vi "SetSyncSettings.vi"(6 "X SyncOut Enabled":bool=TRUE, 7 "Y SyncOut Enabled":bool, 8 "error in (no error)":errorcluster, 9 "Calibration":cluster{dbl, "MicrostepMode":u32}[](array[cluster]), 10 "Step Sizes(mm)":dbl[](array[numeric]), 11 "IDs":i32[](array[numeric])) -> (0 "error out":errorcluster, 3 "IDs Out":i32[](array[numeric]))   [LabVIEW 2020]
uses:
  Sync_outFlags.ctl
  Sync_inFlags.ctl
  libximc.lvlib
panel:
  out "SyncOutPeriod":u32[](array[numeric])
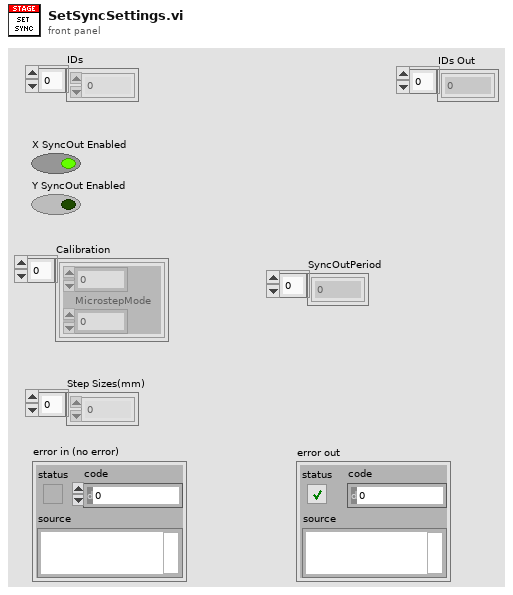
[diagram p1: front panel]
types:
  T1 = cluster{"SyncInFlags":u32, "ClutterTime":u32, "Position":sgl, "Speed":sgl}
  T2 = typedef "Sync_inFlags.ctl" = cluster{"Enabled":bool, "invert":bool, "go_to_position":bool}
  T3 = cluster{"SyncOutFlags":u32, "SyncOutPulseSteps":u32, "SyncOutPeriod":u32, "Accuracy":sgl}
  T4 = typedef "Sync_outFlags.ctl" = cluster{"Enabled":bool, "state":bool, "invert":bool, "in_steps":bool, "on_start":bool, "on_stop":bool, "on_period":bool}
  T5 = cluster{"SyncInFlags":u32, "ClutterTime":u32, "Position":sgl, "Speed":sgl}[]
  T6 = cluster{"SyncOutFlags":u32, "SyncOutPulseSteps":u32, "SyncOutPeriod":u32, "Accuracy":sgl}[]
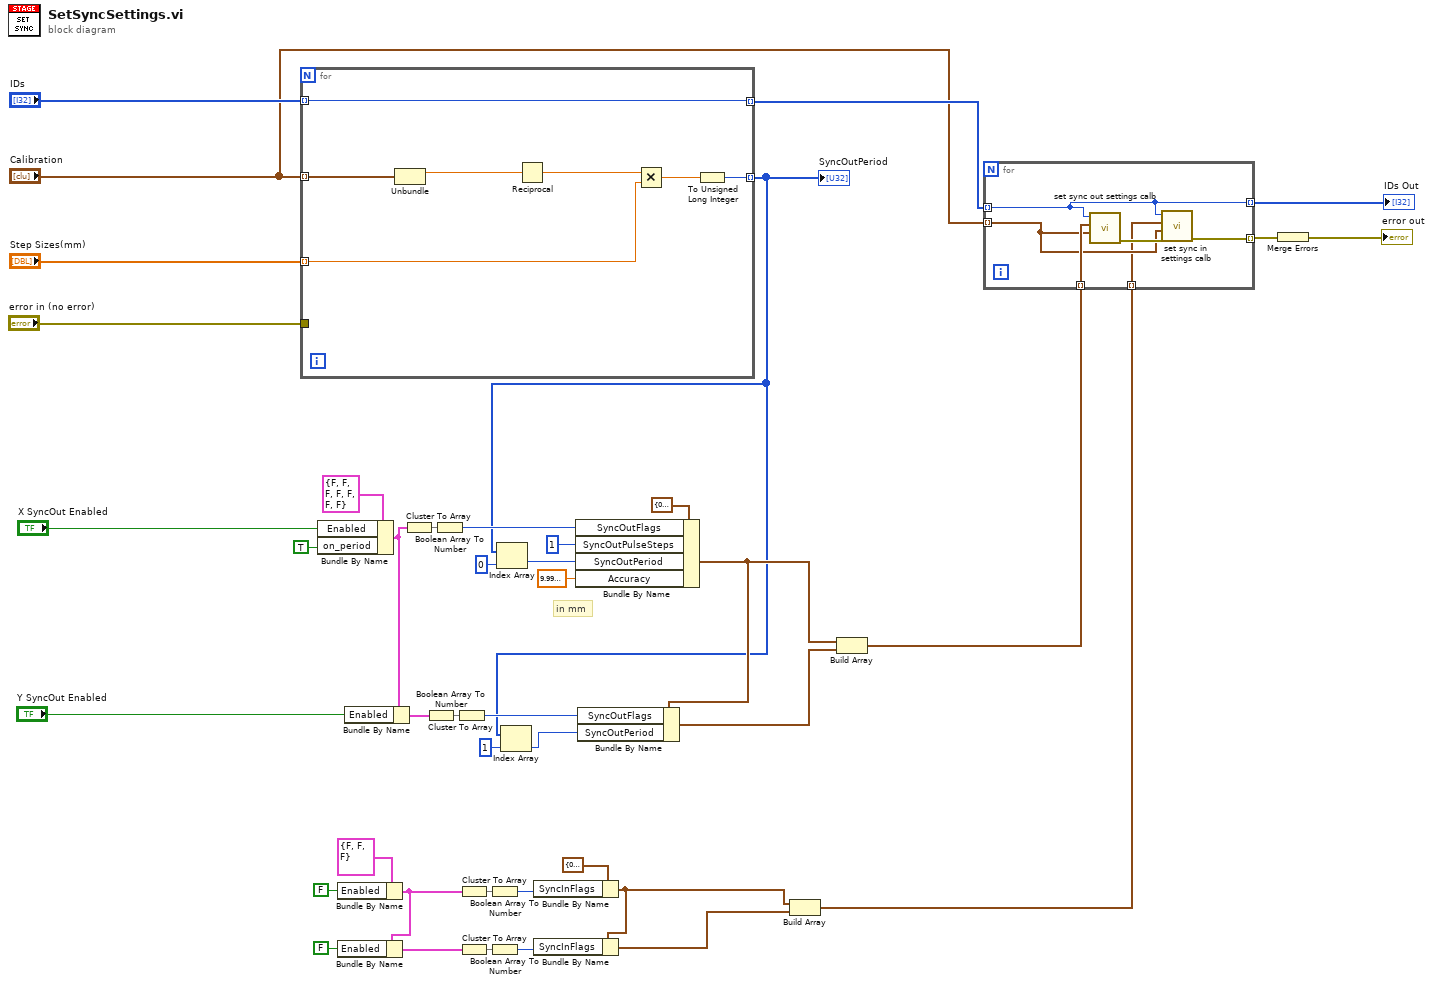
[diagram p0: block diagram]
diagram:
  # "in mm"
  n1 = for {
    tunnel: [w49] -> w21 mode=indexing
    tunnel: "IDs" -> [w49] mode=indexing
    tunnel: "Calibration" -> [w48] mode=indexing
    tunnel: "Step Sizes(mm)" -> [w47] mode=indexing
    tunnel: [w46] -> w22 mode=indexing
    tunnel: "error in (no error)" -> [_]
    n2 = Unbundle(w48) -> (w45:dbl)  [unwired: 1 out]
    n3 = Reciprocal(x=w45) -> (1/x=w44:dbl)
    n4 = Multiply(x=w44, y=w47) -> (x*y=w43:dbl)
    n5 = To Unsigned Long Integer(number=w43) -> (unsigned 32bit integer=w46:u32)
  }
  "SyncOutPeriod" <- w22
  n6 = Bundle By Name(cluster=T4 {"Enabled"=FALSE, "state"=FALSE, "invert"=FALSE, "in_steps"=FALSE, "on_start"=FALSE, "on_stop"=FALSE, "on_period"=FALSE} ("Sync_out Flags"), "Enabled"="X SyncOut Enabled", "on_period"=TRUE) -> (w27:T4)
  n7 = Bundle By Name(cluster=T2 {"Enabled"=FALSE, "invert"=FALSE, "go_to_position"=FALSE} ("Sync_out Flags"), "Enabled"=FALSE) -> (w7:T2)
  n8 = Bundle By Name(cluster=w7, "Enabled"=FALSE) -> (w8:T2)
  n9 = Bundle By Name(cluster=w27, "Enabled"="Y SyncOut Enabled") -> (w35:T4)
  n10 = Cluster To Array(cluster=w27) -> (array=w40:bool[])
  n11 = Cluster To Array(cluster=w35) -> (array=w36:bool[])
  n12 = Boolean Array To Number(Boolean array=w40) -> (number=w39:u32)
  n13 = Boolean Array To Number(Boolean array=w36) -> (number=w37:u32)
  n14 = Cluster To Array(cluster=w7) -> (array=w18:bool[])
  n15 = Cluster To Array(cluster=w8) -> (array=w9:bool[])
  n16 = Boolean Array To Number(Boolean array=w18) -> (number=w17:u32)
  n17 = Boolean Array To Number(Boolean array=w9) -> (number=w10:u32)
  n18 = Index Array(array=w22, index=0) -> (element=w26:u32)
  n19 = Index Array(array=w22, index=1) -> (element=w23:u32)
  n20 = Bundle By Name(cluster=T1 {"SyncInFlags"=0, "ClutterTime"=0, "Position"=0.0, "Speed"=0.0} ("sync_in_settings_calb"), "SyncInFlags"=w17) -> (w6:T1)
  n21 = Bundle By Name(cluster=w6, "SyncInFlags"=w10) -> (w5:T1)
  n22 = Bundle By Name(cluster=T3 {"SyncOutFlags"=0, "SyncOutPulseSteps"=0, "SyncOutPeriod"=0, "Accuracy"=0.0} ("sync_out_settings_calb"), "SyncOutFlags"=w39, "SyncOutPulseSteps"=u32 1, "SyncOutPeriod"=w26, "Accuracy"=sgl 1e-06) -> (w28:T3)
  n23 = Bundle By Name(cluster=w28, "SyncOutFlags"=w37, "SyncOutPeriod"=w23) -> (w34:T3)
  n24 = Build Array(w6, w5) -> (w13:T5)
  n25 = Build Array(w28, w34) -> (w20:T6)
  n26 = for {
    tunnel: w21 -> [w54] mode=indexing
    tunnel: w20 -> [w55] mode=indexing
    tunnel: "Calibration" -> [w51] mode=indexing
    tunnel: [w54] -> w14 mode=indexing
    tunnel: [w52] -> w4 mode=indexing
    tunnel: w13 -> [w50] mode=indexing
    n27 = call "set sync out settings calb.vi"("calibration"=w51, "sync_out_settings_calb"=w55, "id"=w54) -> ("error out"=w53:errorcluster)  [unwired: 7 in, 1 out]
    n28 = call "set sync in settings calb.vi"("error in (no error)"=w53, "calibration"=w51, "sync_in_settings_calb"=w50, "id"=w54) -> ("error out"=w52:errorcluster)  [unwired: 6 in, 1 out]
  }
  "IDs Out" <- w14
  n29 = Merge Errors(w4) -> (→"error out":errorcluster)
